vi "Read Array.vi"(8 "error in (no error)":errorcluster, 11 "Enum in":refnum<class "Enum.lvclass">) -> (0 "error out":errorcluster, 2 "Array":string[](array[string]), 3 "Enum out":refnum<class "Enum.lvclass">)   [LabVIEW 2018, in "Enum.lvclass"]
doc: "Read the array."
uses:
  Enum.lvclass
  Enum.lvclass/Enum.ctl
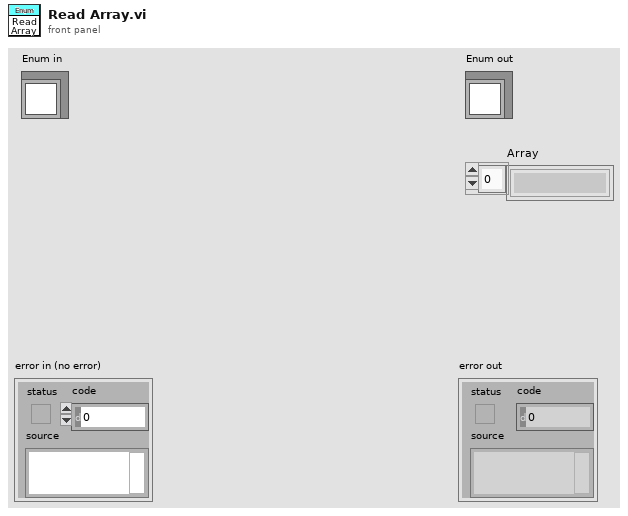
[diagram p1: front panel]
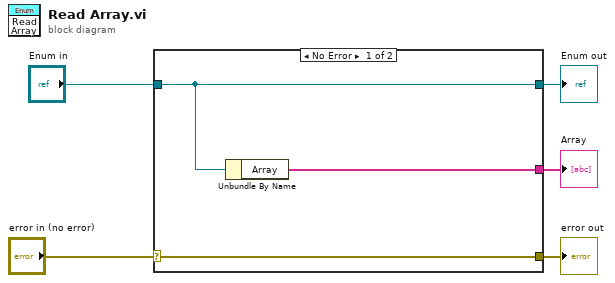
[diagram p0: block diagram]
diagram:
  n1 = case shown="No Error" "error in (no error)" {
    selector: "error in (no error)" -> [w8 w9]
    tunnel: [w8 w9] -> w4
    tunnel: [w7 w10] -> w2
    tunnel: "Enum in" -> [w7 w10]
    tunnel: [w6 _] -> w1
    frame No Error {
      n2 = Unbundle By Name(w7) -> ("Array"=w6:string[])
    }
    frame Error {
    }
  }
  "error out" <- w4
  "Enum out" <- w2
  "Array" <- w1
